vi "set_level.vi"(8 "error in (no error)":errorcluster, 9 "level":T1=200 items=["OFF"=0, "FATAL"=100, "ERROR"=200, "WARN"=300, "INFO"=400, "DEBUG"=500, "TRACE"=600, "ALL"=65535], 11 "Queue Log Provider in":refnum<class "Queue Log Provider.lvclass">) -> (0 "error out":errorcluster, 3 "Queue Log Provider out":refnum<class "Queue Log Provider.lvclass">)   [LabVIEW 2019, in "LVCOOOP.lvlib" / "Utility API.lvlib" / "Queue Log Provider.lvclass"]
uses:
  Queue Log Provider.lvclass
  Log Service/public/level.ctl
  Queue Log Provider.lvclass/Queue Log Provider.ctl
  Log Service/Log Service.lvclass
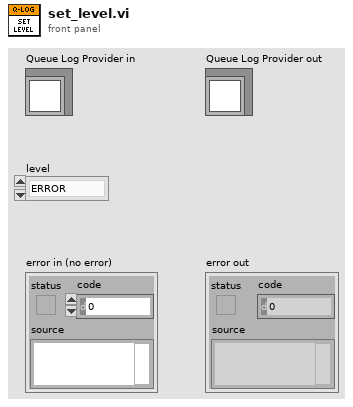
[diagram p1: front panel]
types:
  T1 = typedef "LVCOOOP.lvlib/Utility API.lvlib/Log Service.lvclass/level.ctl" = u16
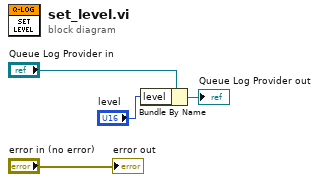
[diagram p0: block diagram]
diagram:
  n1 = Bundle By Name(cluster="Queue Log Provider in", "level"="level") -> (→"Queue Log Provider out":refnum<class "Queue Log Provider.lvclass">)
  "error out" <- "error in (no error)"
